vi "prueba_com.vi"() -> ()   [LabVIEW 2021]
uses:
  <vilib>/MakerHub/LINX/Private/Local IO/LinxI2cWrite.vi
  <vilib>/MakerHub/LINX/Public/Utilities/Check Channel.vi
  <vilib>/MakerHub/LINX/Public/Utilities/Open Serial.vi
  <vilib>/MakerHub/LINX/Private/Utilties/Generate Error.vi
  <vilib>/MakerHub/LINX/LMH-LINX.lvlib
panel:
  out "Array 2":u8[](array[numeric])
  out "Array":string[](array[string])
  in  "Boolean":bool
  out "Device Name 2":string
  out "Error Out 2":errorcluster
  in  "Error In 2":errorcluster
  in  "Serial Port 2":refnum<visa-resource-name>="N/A"
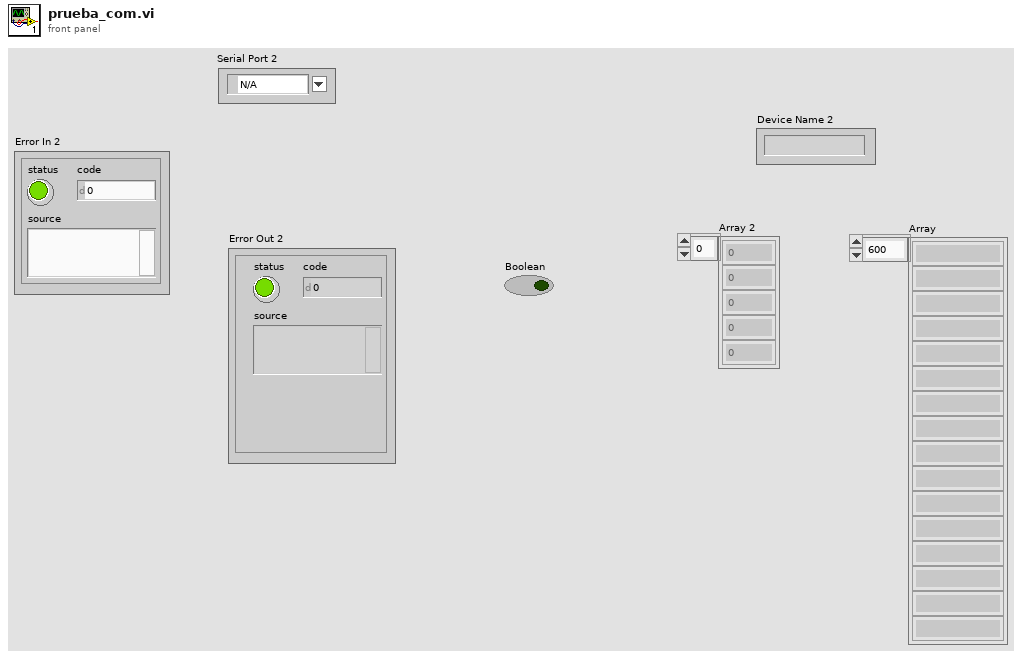
[diagram p1: front panel]
types:
  T1 = typedef "LMH-LINX.lvlib/LINX Ref.ctl" = cluster{"IO":T2, "Interface":T3, "LINX Device Config":T4}
  T2 = typedef "LMH-LINX.lvlib/Platform.ctl" = enum16{"Remote", "Local"}
  T3 = typedef "LMH-LINX.lvlib/Interface.ctl" = enum16{"Serial", "TCP"}
  T4 = typedef "LMH-LINX.lvlib/Device.lvlib/LINX Device Config.ctl" = cluster{"Interface":T3, "COM Port":refnum<visa-resource-name>, "TCP Configuration":T5, "Device Family":u8, "Device ID":u8, "Device Name":string, "TCP Ref":refnum<k5>, "Channels":T6}
  T5 = typedef "LMH-LINX.lvlib/Device.lvlib/TCP Config.ctl" = cluster{"IP Address":string, "Port":u16}
  T6 = typedef "LMH-LINX.lvlib/Channels.ctl" = cluster{"DI":u8[], "DO":u8[], "AI":u8[], "AO":u8[], "PWM":u8[], "QE":u8[], "UART":u8[], "I2C 2":u8[], "SPI":u8[], "CAN":u8[], "Servo":u8[], "AI Ref (V)":dbl, "AI Resolution (Bits)":u8, "AO Ref (V)":dbl, "AO Resolution (Bits)":u8}
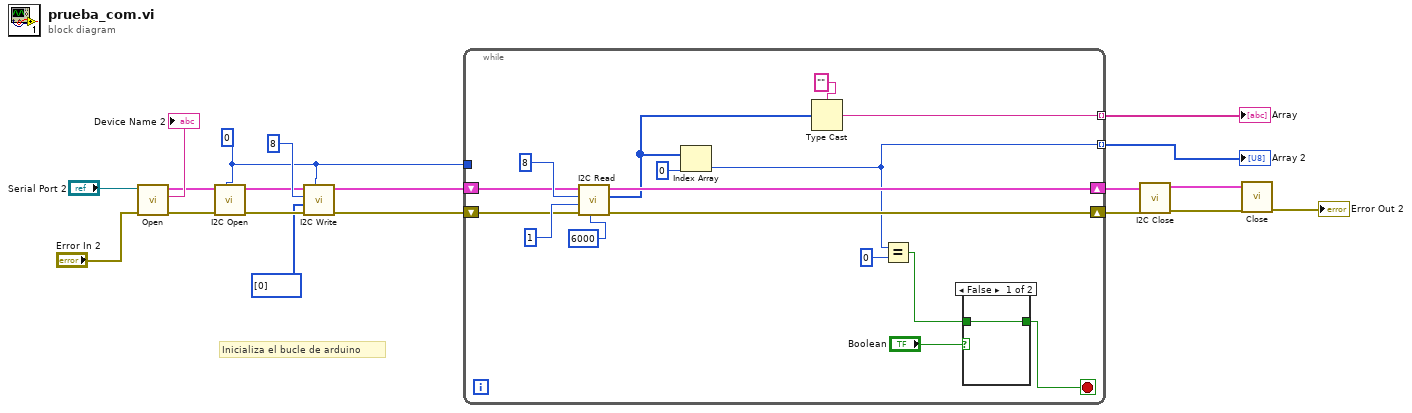
[diagram p0: block diagram]
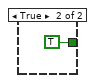
[diagram p2: hidden frame]
diagram:
  w4 = u8 0 ("I2C Channel")
  # "Inicializa el bucle de arduino"
  n1 = call-poly <vilib>:"Open.vi"("Error In"="Error In 2", "Serial Port"="Serial Port 2") -> ("Error Out"=w3:errorcluster, "Device Name"=→"Device Name 2":string, "LINX Resource"=w12:T1)  [unwired: 7 in]
  n2 = call <vilib>:"I2C Open.vi"("I2C Channel (0)"=w4, "Error In"=w3, "LINX Resource"=w12) -> ("Error Out"=w10:errorcluster, "LINX Resource"=w7:T1)  [unwired: 7 in]
  n3 = call <vilib>:"I2C Write.vi"("I2C Channel"=w4, "Error In"=w10, "Data"=u8[] [0], "I2C Slave Address (0)"=u8 8, "LINX Resource"=w7) -> ("Error Out"=w5:errorcluster, "LINX Resource"=w6:T1)  [unwired: 5 in]
  n4 = while {
    tunnel: w4 -> [_]
    shift-right: [w34] -> w14
    shift-left: w5 -> [w28]
    shift-right: [w27] -> w13
    shift-left: w6 -> [w29]
    tunnel: [w24] -> w2 mode=indexing
    tunnel: [w22] -> w1 mode=indexing
    stop <- w21 stop-if-true
    n5 = call <vilib>:"I2C Read.vi"("Timeout (1000 ms)"=u16 6000, "Error In"=w28, "Bytes To Read"=u8 1, "I2C Slave Address (0)"=u8 8, "LINX Resource"=w29) -> ("Error Out"=w34:errorcluster, "Data"=w26:u8[], "LINX Resource"=w27:T1)  [unwired: 4 in]
    n6 = Index Array(array=w26, index=0) -> (element=w22:u8)
    n7 = Type Cast(type="", x=w26) -> (*(type *) &x=w24:string)
    n8 = Equal?(x=w22, y=u8 0) -> (x = y?=w31:bool)
    n9 = case shown="False" "Boolean" {
      tunnel: w31 -> [w36 _]
      tunnel: [w36 TRUE] -> w21
      frame False {
      }
      frame True {
      }
    }
  }
  "Array" <- w2
  "Array 2" <- w1
  n10 = call <vilib>:"I2C Close.vi"("Error In"=w14, "LINX Resource"=w13) -> ("Error Out"=w18:errorcluster, "LINX Resource"=w17:T1)  [unwired: 8 in]
  n11 = call <vilib>:"Close.vi"("Error In"=w18, "LINX Resource"=w17) -> ("Error Out"=→"Error Out 2":errorcluster)  [unwired: 9 in]
